vi "Notebook Find String after.vi"(8 "error in (no error)":errorcluster, 9 "After position":i32, 10 "Search String":string, 11 ".NET Refnum in":refnum<k24>) -> (0 "error out":errorcluster, 1 "Location after string":i32, 2 "String location":i32, 3 ".NET Refnum out":refnum<k24>)   [LabVIEW 2021, in "Notebook.lvlib"]
uses:
  Notebook.lvlib
  System.Windows.Forms
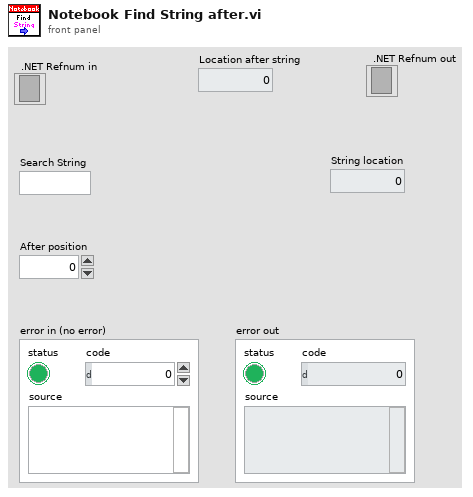
[diagram p1: front panel]
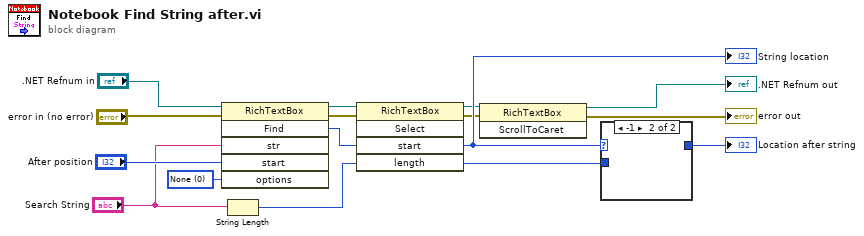
[diagram p0: block diagram]
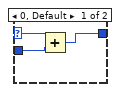
[diagram p2: hidden frame]
diagram:
  w14 = 0 items=["None"=0, "WholeWord"=2, "MatchCase"=4, "NoHighlight"=8, "Reverse"=16] ("options")
  n1 = invoke class="RichTextBox" method="Find"(reference=".NET Refnum in", error in="error in (no error)", "str"="Search String", "start"="After position", "options"=w14) -> (reference out=w6:refnum<k24>, error out=w7:errorcluster, "Find"=w8:i32)  [unwired: 1 in, 3 out]
  "String location" <- w8
  n2 = String Length(string="Search String") -> (length=w13:i32)
  n3 = invoke class="RichTextBox" method="Select"(reference=w6, error in=w7, "start"=w8, "length"=w13) -> (reference out=w4:refnum<k24>, error out=w3:errorcluster)  [unwired: 1 in, 3 out]
  n4 = invoke class="RichTextBox" method="ScrollToCaret"(reference=w4, error in=w3) -> (reference out=→".NET Refnum out":refnum<k24>, error out=→"error out":errorcluster)  [unwired: 1 in, 1 out]
  n5 = case shown="-1" w8 {
    selector: w8 -> [w17 _]
    tunnel: [w16 _] -> w9
    tunnel: w13 -> [w15 _]
    frame 0, Default {
      n6 = Add(x=w17, y=w15) -> (x+y=w16:i32)
    }
    frame -1 {
    }
  }
  "Location after string" <- w9
